vi "macro_MecaDriveOdomUpdate.vi"   [LabVIEW 2019, in "Trajectory_Library.lvlib"]
uses:
  Trajectory_Library.lvlib
types:
  T1 = typedef "Trajectory_Library.lvlib/MECA_WHEEL_POSITIONS.ctl" = cluster{"FrontLeft":dbl, "FrontRight":dbl, "RearLeft":dbl, "RearRight":dbl, "P":bool}
  T2 = typedef "Trajectory_Library.lvlib/ROTATION2D.ctl" = cluster{"VALUE":dbl, "COS":dbl, "SIN":dbl}
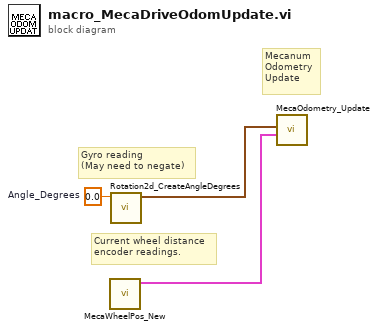
[diagram p0: block diagram]
diagram:
  w3 = 0.0  # Angle_Degrees
  # "Mecanum\nOdometry\nUpdate"
  # "Current wheel distance\nencoder readings."
  # "Gyro reading\n(May need to negate)"
  n1 = call "MecaWheelPos_New.vi"() -> ("MECA_WHEEL_POSITIONS"=w1:T1)  [unwired: 11 in]
  n2 = call "Rotation2d_CreateAngleDegrees.vi"("Angle_Degrees"=w3) -> ("ROTATION"=w2:T2)  [unwired: 10 in]
  n3 = call "MecaOdometry_Update.vi"("WheelPosition"=w1, "GyroAngle"=w2) -> ()  [unwired: 8 in, 2 out]
